vi "appControlView.vi"(10 "UserEvents in":refnum<class "UserEvents.lvclass">) -> ()   [LabVIEW 2013, in "ILCBTViews.lvlib"]
uses:
  ILCBTViews.lvlib
  UserEvents/UserEvents.lvclass
  CommandFactory/CommandFactory.lvclass
  UserEvents/UserEvents.lvclass/UserEvents.ctl
  Typedefs/StateSelector.ctl
  Typedefs/CommandSelector.ctl
  Typedefs/ILCBTTypedefs.lvlib
panel:
  in  "goToStandbyIsTrue":bool
  in  "clearErrorIsTrue":bool
  in  "exitIsTrue":bool
  in  "startIsTrue":bool
types:
  T1 = typedef "ILCBTTypedefs.lvlib/PubDataEvents.ctl" = cluster{"State":refnum<user-event>, "ErrorCode":refnum<user-event>, "OutputData":refnum<user-event>, "LogPath":refnum<user-event>}
  T2 = typedef "ILCBTTypedefs.lvlib/SubDataEvents.ctl" = cluster{"Command":refnum<user-event>}
  T3 = cluster{"Event Registration Refnum":refnum<event-registration>}
  T4 = typedef "ILCBTTypedefs.lvlib/StateSelector.ctl" = enum16{"EnabledState", "FaultState", "OffState", "StandbyState"}
  T5 = typedef "ILCBTTypedefs.lvlib/CommandSelector.ctl" = enum16{"ClearError", "Exit", "StandBy", "Start", "Update"}
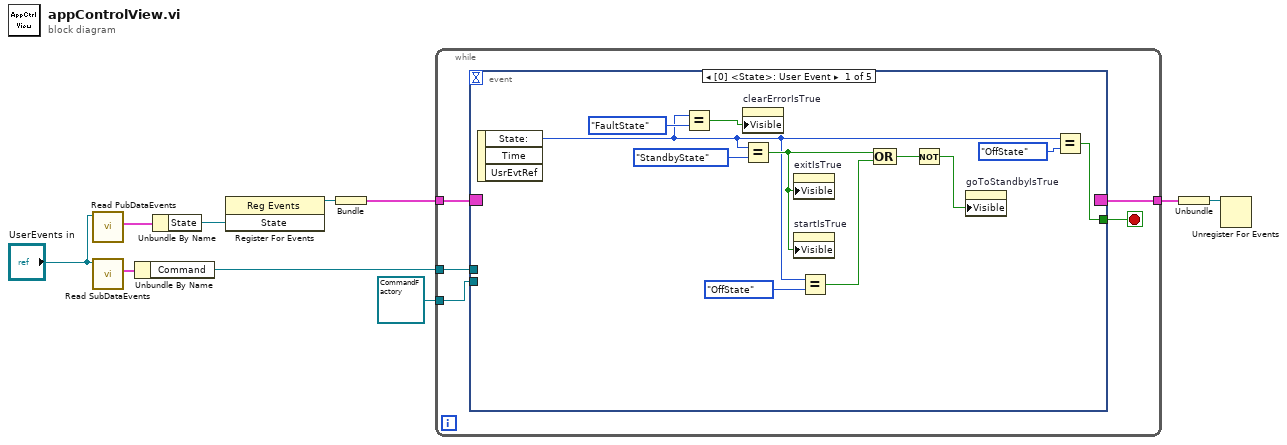
[diagram p0: block diagram]
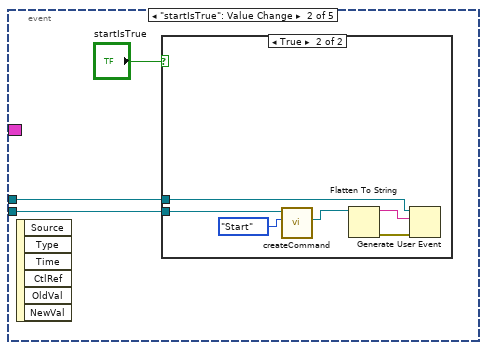
[diagram p2: hidden frame]
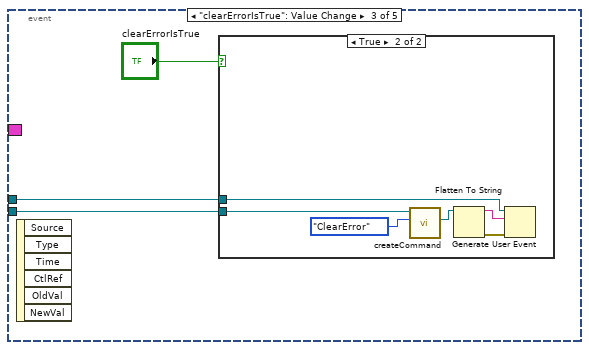
[diagram p4: hidden frame]
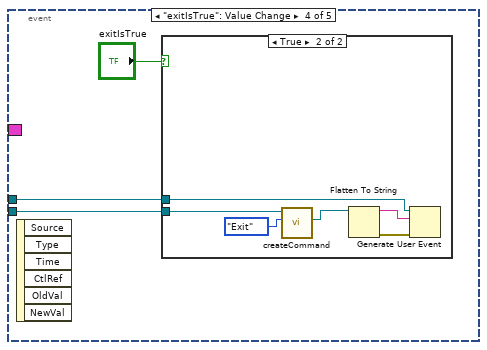
[diagram p6: hidden frame]
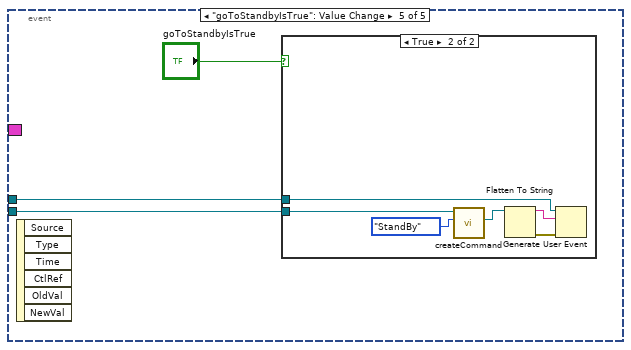
[diagram p8: hidden frame]
diagram:
  n1 = call "Read PubDataEvents.vi"("UserEvents in"="UserEvents in") -> ("PubDataEvents"=w7:T1)  [unwired: 9 in, 1 out]
  n2 = call "Read SubDataEvents.vi"("UserEvents in"="UserEvents in") -> ("SubDataEvents"=w8:T2)  [unwired: 9 in, 1 out]
  n3 = Unbundle By Name(w8) -> ("Command"=w5:refnum<user-event>)
  n4 = Unbundle By Name(w7) -> ("State"=w9:refnum<user-event>)
  n5 = register-events(w9) -> (reference out=w10:refnum<event-registration>)  [unwired: 2 in, 1 out]
  n6 = Bundle("Event Registration Refnum"=w10) -> (w6:T3)  [unwired: 1 in]
  n7 = while {
    tunnel: w6 -> [w15]
    tunnel: w5 -> [w14]
    tunnel: [w13] -> w4
    tunnel: refnum<class "CommandFactory.lvclass"> refnum ("CommandFactory.lvclass") -> [w11]
    stop <- w12 stop-if-true
    n8 = event shown="[0] <State>: User Event" {
      selector: w15 -> [_ _ _ _ _]
      dyn-events: [_ _ _ _ _] -> w13
      timeout: _ -> [_ _ _ _ _]
      tunnel: w14 -> [_ w29 w37 w46 w55]
      tunnel: [w25 _ _ _ _] -> w12
      tunnel: w11 -> [_ w28 w38 w47 w56]
      event User Event {
        n9 = event-data() -> ("State:"=w17:T4)  [unwired: 1 in, 2 out]
        n10 = Equal?(x=w17, y=StateSelector."FaultState") -> (x = y?=w16:bool)
        n11 = property on="clearErrorIsTrue" class="Bool"("Visible"=w16) -> ()  [unwired: 2 in, 2 out]
        n12 = Equal?(x=w17, y=StateSelector."StandbyState") -> (x = y?=w22:bool)
        n13 = property on="exitIsTrue" class="Bool"("Visible"=w22) -> ()  [unwired: 2 in, 2 out]
        n14 = property on="startIsTrue" class="Bool"("Visible"=w22) -> ()  [unwired: 2 in, 2 out]
        n15 = Equal?(x=w17, y=StateSelector."OffState") -> (x = y?=w19:bool)
        n16 = Compound Arithmetic op=OR(w22, w19) -> (w21:bool)
        n17 = Not(x=w21) -> (.not. x?=w20:bool)
        n18 = property on="goToStandbyIsTrue" class="Bool"("Visible"=w20) -> ()  [unwired: 2 in, 2 out]
        n19 = Equal?(x=w17, y=StateSelector."OffState") -> (x = y?=w25:bool)
      }
      event "startIsTrue": Value Change {
        n20 = event-data() -> ()  [unwired: 1 in, 6 out]
        n21 = case shown="True" "startIsTrue" {
          tunnel: w28 -> [_ w35]
          tunnel: w29 -> [_ w31]
          frame False {
          }
          frame True {
            n22 = call-dynamic "createCommand.vi"("Command"=CommandSelector."Start", "CommandFactory in"=w35) -> ("command"=w30:refnum<class "Command.lvclass">)  [unwired: 7 in, 2 out]
            n23 = Flatten To String(anything=w30) -> (data string=w32:string, error out=w33:errorcluster)  [unwired: 3 in, 1 out]
            n24 = Generate User Event(user event=w31, event data cluster=w32, error in=w33) -> ()  [unwired: 1 in, 2 out]
          }
        }
      }
      event "clearErrorIsTrue": Value Change {
        n25 = event-data() -> ()  [unwired: 1 in, 6 out]
        n26 = case shown="True" "clearErrorIsTrue" {
          tunnel: w38 -> [_ w44]
          tunnel: w37 -> [_ w40]
          frame False {
          }
          frame True {
            n27 = call-dynamic "createCommand.vi"("Command"=CommandSelector."ClearError", "CommandFactory in"=w44) -> ("command"=w39:refnum<class "Command.lvclass">)  [unwired: 7 in, 2 out]
            n28 = Flatten To String(anything=w39) -> (data string=w41:string, error out=w42:errorcluster)  [unwired: 3 in, 1 out]
            n29 = Generate User Event(user event=w40, event data cluster=w41, error in=w42) -> ()  [unwired: 1 in, 2 out]
          }
        }
      }
      event "exitIsTrue": Value Change {
        n30 = event-data() -> ()  [unwired: 1 in, 6 out]
        n31 = case shown="True" "exitIsTrue" {
          tunnel: w47 -> [_ w53]
          tunnel: w46 -> [_ w49]
          frame False {
          }
          frame True {
            n32 = call-dynamic "createCommand.vi"("Command"=CommandSelector."Exit", "CommandFactory in"=w53) -> ("command"=w48:refnum<class "Command.lvclass">)  [unwired: 7 in, 2 out]
            n33 = Flatten To String(anything=w48) -> (data string=w50:string, error out=w51:errorcluster)  [unwired: 3 in, 1 out]
            n34 = Generate User Event(user event=w49, event data cluster=w50, error in=w51) -> ()  [unwired: 1 in, 2 out]
          }
        }
      }
      event "goToStandbyIsTrue": Value Change {
        n35 = event-data() -> ()  [unwired: 1 in, 6 out]
        n36 = case shown="True" "goToStandbyIsTrue" {
          tunnel: w56 -> [_ w62]
          tunnel: w55 -> [_ w58]
          frame False {
          }
          frame True {
            n37 = call-dynamic "createCommand.vi"("Command"=CommandSelector."StandBy", "CommandFactory in"=w62) -> ("command"=w57:refnum<class "Command.lvclass">)  [unwired: 7 in, 2 out]
            n38 = Flatten To String(anything=w57) -> (data string=w59:string, error out=w60:errorcluster)  [unwired: 3 in, 1 out]
            n39 = Generate User Event(user event=w58, event data cluster=w59, error in=w60) -> ()  [unwired: 1 in, 2 out]
          }
        }
      }
    }
  }
  n40 = Unbundle(w4) -> ("Event Registration Refnum"=w3:refnum<event-registration>)
  n41 = Unregister For Events(event registration refnum=w3) -> ()  [unwired: 1 in, 1 out]
